vi "FreqRep.vi"(9 "Array":dbl[](array[numeric]), 10 "Numeric":i32) -> (2 "Array 2":dbl[](array[numeric]))   [LabVIEW 2017, in "Andeen-Hagerling 2700.lvlib"]
uses:
  <instrlib>/Andeen-Hagerling 2700/Andeen-Hagerling 2700.lvlib
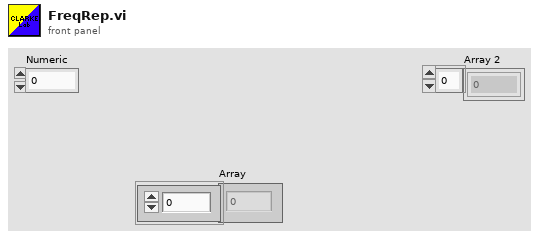
[diagram p1: front panel]
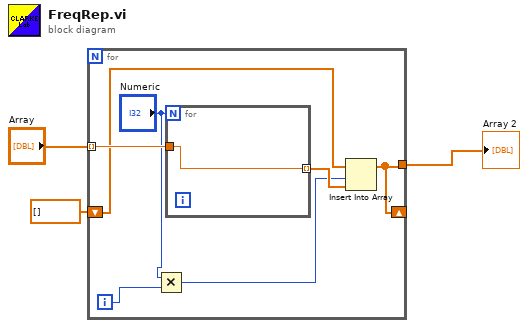
[diagram p0: block diagram]
diagram:
  n1 = for {
    tunnel: "Array" -> [w10] mode=indexing
    tunnel: [w7] -> w2
    shift-right: [w7] -> _
    shift-left: dbl[] [] -> [w8]
    i -> [w5]
    n2 = Multiply(x="Numeric", y=w5) -> (x*y=w4:i32)
    n3 = for {
      N: "Numeric" -> [_]
      tunnel: w10 -> [w11]
      tunnel: [w11] -> w9 mode=indexing
    }
    n4 = Insert Into Array(array=w8, index=w4, new element=w9) -> (w7:dbl[])
  }
  "Array 2" <- w2
